vi "Create FP Item.vi"(6 "Cluster Component":bool, 8 "error in (no error)":errorcluster, 10 "GObject In":refnum<vi>, 11 "GBoolean in":refnum<class "Boolean.lvclass">) -> (0 "error out":errorcluster, 1 "Is Control":bool, 2 "Is Indicator":bool, 3 "GBoolean out":refnum<class "Boolean.lvclass">, 4 "All Objects Created":refnum<class "Object.lvclass">[](array[class]), 5 "Is Visible":bool)   [LabVIEW 2017, in "Front Panel Publisher.lvlib" / "Boolean.lvclass"]
uses:
  Boolean.lvclass
  Control_class/Control.lvclass
  Text_class/Text.lvclass
  Text_class/Enum - Create Text Method.ctl
  Object_class/Object.lvclass
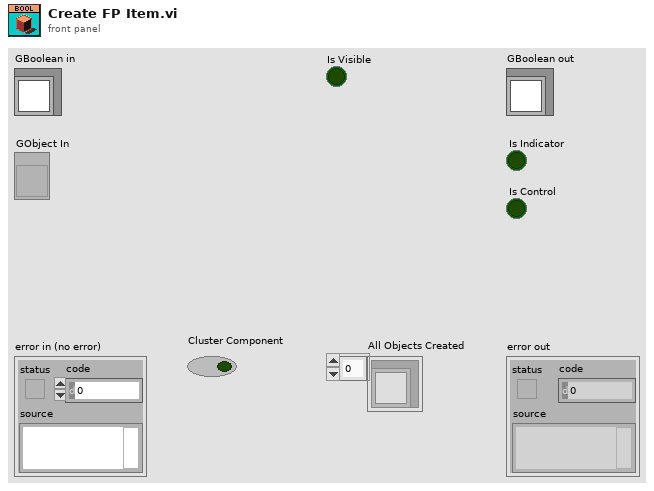
[diagram p1: front panel]
types:
  T1 = typedef "Front Panel Publisher.lvlib/Text.lvclass/Enum - Create Text Method.ctl" = enum16{"Text", "Label", "Caption", "Boolean Text"}
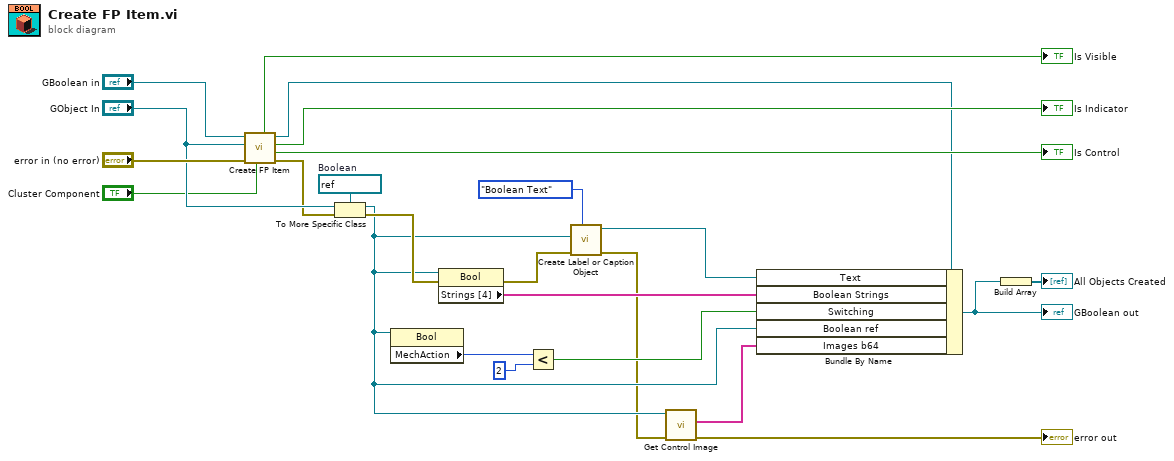
[diagram p0: block diagram]
diagram:
  w18 = refnum<vi> refnum  # Boolean
  n1 = call-parent "Create FP Item.vi"("Cluster Component"="Cluster Component", "error in (no error)"="error in (no error)", "GObject In"="GObject In", "GControl in"="GBoolean in") -> ("error out"=w5:errorcluster, "Is Control"=→"Is Control":bool, "Is Indicator"=→"Is Indicator":bool, "GControl out"=w22:refnum<class "Boolean.lvclass">, "Is Visible"=→"Is Visible":bool)  [unwired: 2 in, 1 out]
  n2 = To More Specific Class(target class=w18, reference="GObject In", error in=w5) -> (specific class reference=w8:refnum<vi>, error out=w16:errorcluster)
  n3 = property class="Bool"(reference=w8) -> ("MechAction"=w15:u32)  [unwired: 1 in, 2 out]
  n4 = property class="Bool"(reference=w8, error in=w16) -> (error out=w9:errorcluster, "Strings [4]"=w13:string[])  [unwired: 1 out]
  n5 = Less?(x=w15, y=u32 2) -> (x < y?=w12:bool)
  n6 = call "Create Label or Caption Object.vi"("Text Type"=Enum_-_Create_Text_Method."Boolean Text", "error in (no error)"=w9, "GObject"=w8) -> ("error out"=w6:errorcluster, "Text out"=w7:refnum<class "Text.lvclass">)  [unwired: 7 in]
  n7 = call "Get Control Image.vi"("error in (no error)"=w6, "Control ref"=w8) -> ("error out"=→"error out":errorcluster, "All base64 Images"=w11:string[])  [unwired: 7 in, 1 out]
  n8 = Bundle By Name(cluster=w22, "Text"=w7, "Boolean Strings"=w13, "Switching"=w12, "Boolean ref"=w8, "Images b64"=w11) -> (w3:refnum<class "Boolean.lvclass">)
  "GBoolean out" <- w3
  n9 = Build Array(w3) -> (→"All Objects Created":refnum<class "Boolean.lvclass">[])
